vi "Obtain Broadcast Events for Registration.vi"(8 "error in":errorcluster) -> (0 "error out":errorcluster, 2 "Already running?":bool, 3 "Panther Dashboard Broadcast Events":T1)   [LabVIEW 2019, in "Panther Dashboard.lvlib"]
doc: "Return the broadcast event refnums so the module's caller can register for the module's broadcast events.\n_____\nBased on DQMH Project Template 6.1.0.94."
uses:
  Panther Dashboard.lvlib
  Broadcast Events--cluster.ctl
  Did Init Argument--cluster.ctl
  Status Updated Argument--cluster.ctl
  Error Reported Argument--cluster.ctl
  Stop Argument--cluster.ctl
  Get Module Execution Status Argument--cluster.ctl
  References Updated Argument--cluster.ctl
  Module type--enum.ctl
  Progress updated Argument--cluster.ctl
  Scale Updated Argument--cluster.ctl
  Connector Pane Updated Argument--cluster.ctl
  Documentation Updated Argument--cluster.ctl
  Documentation--cluster.ctl
  Module Type Updated Argument--cluster.ctl
  Theme Updated Argument--cluster.ctl
  Project Description Updated Argument--cluster.ctl
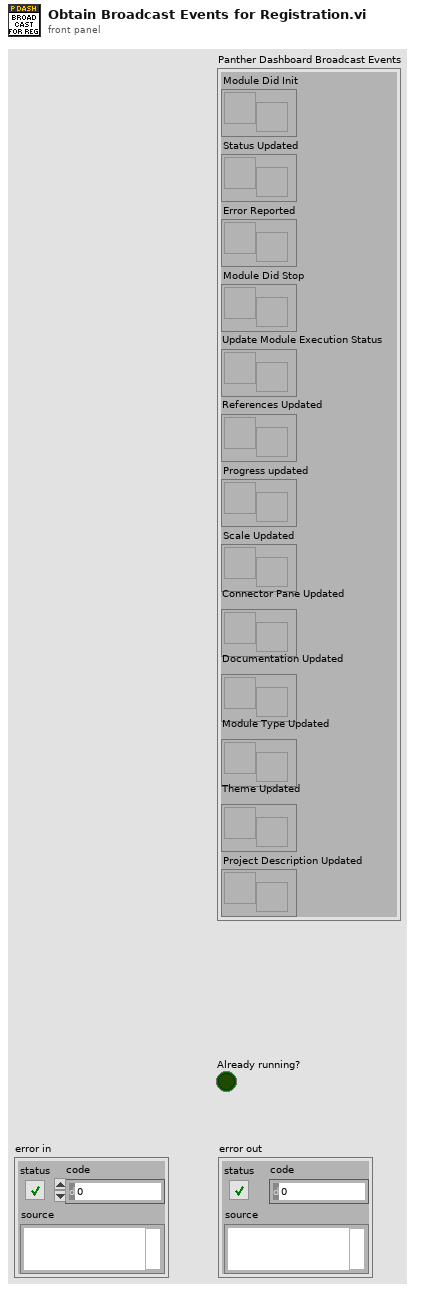
[diagram p1: front panel]
types:
  T1 = typedef "Panther Dashboard.lvlib/Broadcast Events--cluster.ctl" = cluster{"Module Did Init":refnum<user-event>, "Status Updated":refnum<user-event>, "Error Reported":refnum<user-event>, "Module Did Stop":refnum<user-event>, "Update Module Execution Status":refnum<user-event>, "References Updated":refnum<user-event>, "Progress updated":refnum<user-event>, "Scale Updated":refnum<user-event>, "Connector Pane Updated":refnum<user-event>, "Documentation Updated":refnum<user-event>, "Module Type Updated":refnum<user-event>, "Theme Updated":refnum<user-event>, "Project Description Updated":refnum<user-event>}
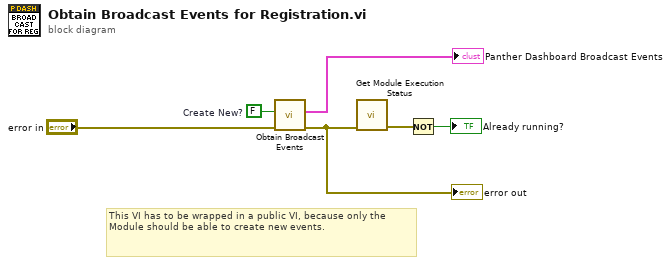
[diagram p0: block diagram]
diagram:
  w3 = FALSE  # Create New?
  # "This VI has to be wrapped in a public VI, because only the Module should be able to create new events."
  n1 = call "Obtain Broadcast Events.vi"("error in"="error in", "Create New? (F)"=w3) -> ("error out"=w5:errorcluster, "Panther Dashboard Broadcast Events"=→"Panther Dashboard Broadcast Events":T1)  [unwired: 8 in]
  "error out" <- w5
  n2 = call "Get Module Execution Status.vi"("error in (no error)"=w5) -> ("error out"=w4:errorcluster)  [unwired: 10 in]
  n3 = Not(x=w4) -> (.not. x?=→"Already running?":bool)
